vi "initialize_data_log.vi"(7 "Overwrite?":bool, 8 "error in (no error)":errorcluster, 9 "Initialization Data":variant, 10 "Path":path, 11 "lfield_logger in":refnum<class "lfield_logger.lvclass">) -> (0 "error out":errorcluster, 3 "lfield_logger out":refnum<class "lfield_logger.lvclass">)   [LabVIEW 2015, in "lfield_logger.lvclass"]
uses:
  lfield_logger.lvclass
  lfield_logger.lvclass/lfield_logger.ctl
  <vilib>/UPVI/lvhdf5/file.llb/LVH5F Operation.ctl
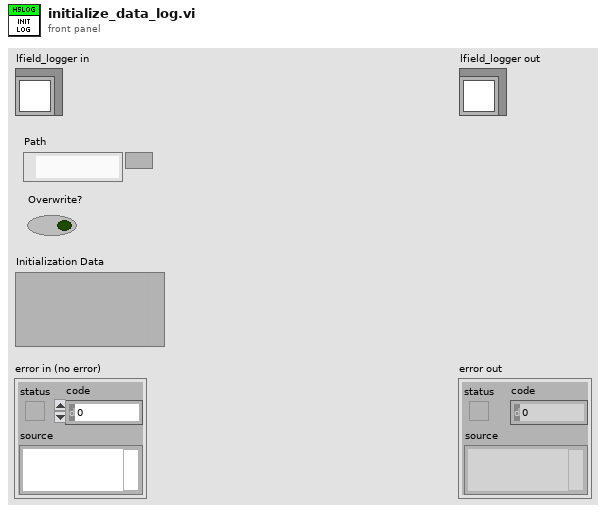
[diagram p1: front panel]
types:
  T1 = typedef "LVH5F Operation.ctl" = enum16{"open", "open or create", "create or replace", "create or replace (with confirmation)", "create", "open (read only)"}
  T2 = typedef "HDF5 Ref.ctl" = refnum<k1>
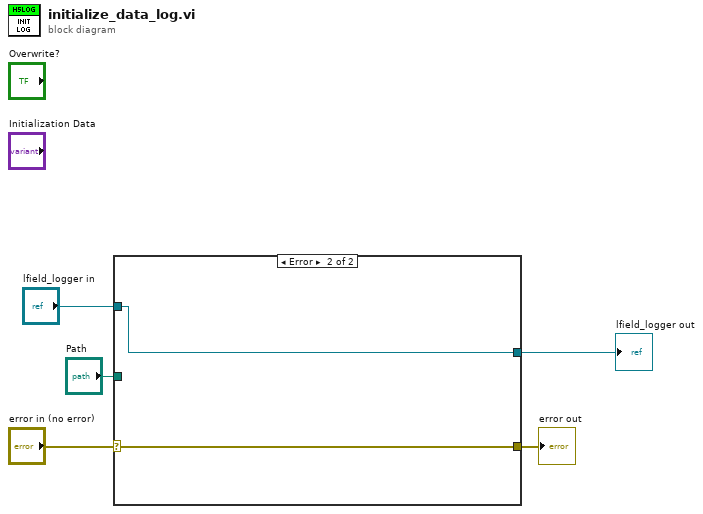
[diagram p0: block diagram]
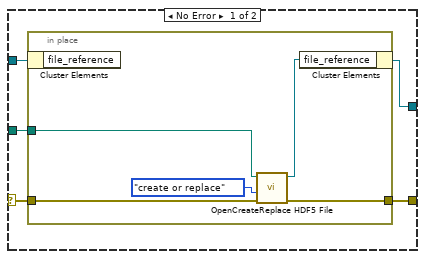
[diagram p2: hidden frame]
diagram:
  n1 = case shown="Error" "error in (no error)" {
    selector: "error in (no error)" -> [w9 w17]
    tunnel: "Path" -> [w10 _]
    tunnel: "lfield_logger in" -> [w8 w16]
    tunnel: [w7 w17] -> w2
    tunnel: [w6 w16] -> w1
    frame No Error {
      n2 = in-place {
        in-place-border: w10 -> [w15]
        in-place-border: w9 -> [w13]
        in-place-border: [w11] -> w7
        n3 = in-place-cluster #1(w8) -> ()  [unwired: 1 out]
        n4 = call <vilib>:"OpenCreateReplace HDF5 File.vi"("error in (no error)"=w13, "function (open or create)"=LVH5F_Operation."create or replace", "path"=w15) -> ("error out"=w11:errorcluster, "HDF5 Ref out"=w12:T2)  [unwired: 5 in]
        n5 = in-place-cluster #1("file_reference"=w12) -> (w6:refnum<class "lfield_logger.lvclass">)
      }
    }
    frame Error {
    }
  }
  "error out" <- w2
  "lfield_logger out" <- w1
